vi "firstCallTest.vi"(8 "error in (no error)":errorcluster, 10 "firstCall":bool=TRUE, 11 "Utilities in":refnum<class "Utilities.lvclass">) -> (0 "error out":errorcluster, 1 "index of element":i32, 2 "firstCallArray":bool[](array[boolean]), 3 "Utilities out":refnum<class "Utilities.lvclass">)   [LabVIEW 2023, in "Utilities.lvclass"]
uses:
  Utilities.lvclass
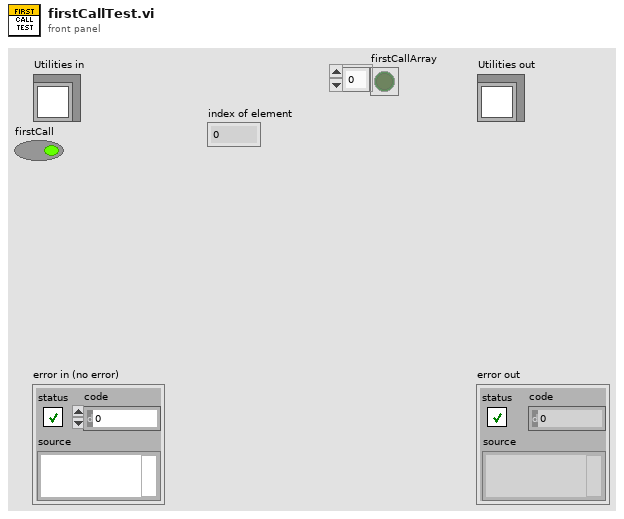
[diagram p1: front panel]
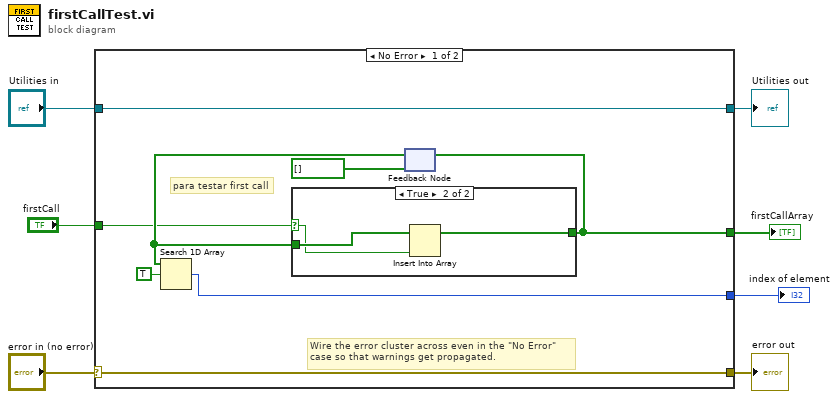
[diagram p0: block diagram]
diagram:
  n1 = case shown="No Error" "error in (no error)" {
    selector: "error in (no error)" -> [w14 w21]
    tunnel: [w14 w21] -> w6
    tunnel: [w15 w20] -> w4
    tunnel: "Utilities in" -> [w15 w20]
    tunnel: "firstCall" -> [w10 _]
    tunnel: [w9 _] -> w2
    tunnel: [w8 _] -> w1
    frame No Error {
      # "para testar first call"
      # "Wire the error cluster across even in the \"No Error\"\ncase so that warnings get propagated."
      n2 = feedback #1(bool[] []) -> (w12:bool[])
      n3 = Search 1D Array(1D array=w12, element=TRUE) -> (index of element=w8:i32)  [unwired: 1 in]
      n4 = case shown="True" w10 {
        selector: w10 -> [_ w17]
        tunnel: w12 -> [w16 w19]
        tunnel: [w16 w18] -> w9
        frame False {
        }
        frame True {
          n5 = Insert Into Array(array=w19, new element=w17) -> (w18:bool[])  [unwired: 1 in]
        }
      }
      n6 = feedback-in #1(w9) -> ()
    }
    frame Error {
    }
  }
  "error out" <- w6
  "Utilities out" <- w4
  "firstCallArray" <- w2
  "index of element" <- w1
